vi "Problem 5.vi"() -> (3 "Smallest Divisible 1-20":u64)   [LabVIEW 2013, in "Problem 5.lvlib"]
uses:
  Problem 5.lvlib
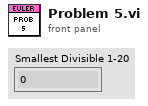
[diagram p1: front panel]
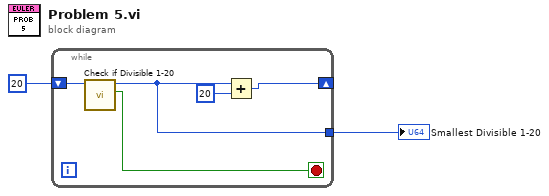
[diagram p0: block diagram]
diagram:
  n1 = while {
    shift-right: [w3] -> _
    shift-left: u64 20 -> [w7]
    tunnel: [w4] -> w1
    stop <- w5 stop-if-true
    n2 = call "Check if Divisible 1-20.vi"("Number to Test?"=w7) -> ("Passed?"=w5:bool, "Number Tested"=w4:u64)  [unwired: 9 in]
    n3 = Add(x=w4, y=u64 20) -> (x+y=w3:u64)
  }
  "Smallest Divisible 1-20" <- w1
